vi "Check For Last Winner Board.vi"(8 "Matrixes Status In":bool[][][](array[boolean]), 10 "Turn Number":i32, 11 "Boards":i32[][][](array[numeric])) -> (0 "Matrixes Status Out":bool[][][](array[boolean]), 1 "Winner Board Status":bool[][](array[boolean]), 2 "Winner Board":i32[][](array[numeric]), 3 "Boards Without Winner":i32[][][](array[numeric]))   [LabVIEW 2019, in "Day 4.lvlib"]
uses:
  Day 4.lvlib
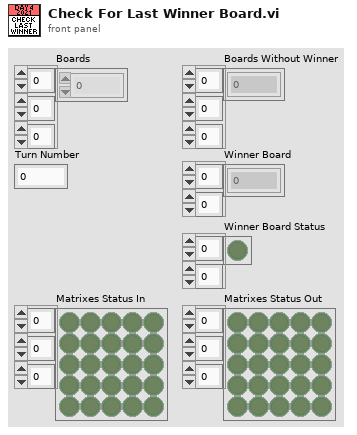
[diagram p1: front panel]
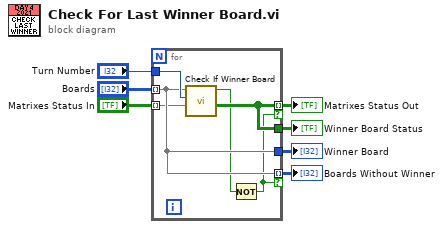
[diagram p0: block diagram]
diagram:
  n1 = for {
    tunnel: "Boards" -> [w11] mode=indexing
    tunnel: "Turn Number" -> [w13]
    tunnel: [w12] -> w5 mode=indexing if=w8
    tunnel: "Matrixes Status In" -> [w10] mode=indexing
    tunnel: [w12] -> w3
    tunnel: [w11] -> w2
    tunnel: [w11] -> w1 mode=indexing if=w8
    n2 = call "Check If Winner Board.vi"("Matriz Status In"=w10, "Turn Number"=w13, "Boards"=w11) -> ("Matriz Status Out"=w12:bool[][], "Winner?"=w9:bool)  [unwired: 7 in]
    n3 = Not(x=w9) -> (.not. x?=w8:bool)
  }
  "Matrixes Status Out" <- w5
  "Winner Board Status" <- w3
  "Winner Board" <- w2
  "Boards Without Winner" <- w1
